vi "UDP_Stream(DMA).vi"() -> ()   [LabVIEW 2015]
uses:
  <vilib>/Platform/TimedLoop/XDataNode/timing_clust.ctl
  <vilib>/Platform/TimedLoop/XDataNode/nitl_modes.ctl
  <vilib>/Platform/TimedLoop/XDataNode/wakeup.ctl
  <vilib>/FPGAPlugInAG/cRIO-9063/niLvFpga_Open_cRIO-9063.vi
  <vilib>/rvi/interface/common/dynamic/niFpgaDynamicAddResources.vi
  <vilib>/Utility/error.llb/Error Cluster From Error Code.vi
  <vilib>/rvi/errors/niLvFpgaAdjustHostInterfaceError.vi
  <vilib>/Platform/TimedLoop/XDataNode/loadnilvce.vi
  <vilib>/rvi/interface/nirviOpenFPGA/nirviOpenFPGA.xnode
  FPGA Bitfiles/VCU-VEHICLEMODEL_FPGATarget_CANBasic(FPGA)_WVt1gIpoBPw.lvbitx
  Basic (FPGA) CAN Engine .vi
  <vilib>/rvi/interface/nirviReadWriteControl/nirviReadWriteControl.xnode
  <vilib>/Platform/TimedLoop/XDataNode/XDataNode.xnode
  <vilib>/Platform/TimedLoop/XDataNode/XDNodeRunTimeDep.lvlib
  NiFpgaLv.dll
  <vilib>/rvi/interface/Simulation/niFpgaSimulationCallBeginRW.vi
panel:
  out "Inbound Data String":string
  in  "Stop":bool
  out "CAN1 Data String":string
  out "CAN0 Data String":string
  out "CAN1-Time":u64
  out "CAN1-OldTime":u64
  out "CAN0-OldTime":u64
  out "CAN0-Time":u64
  in  "Start":bool
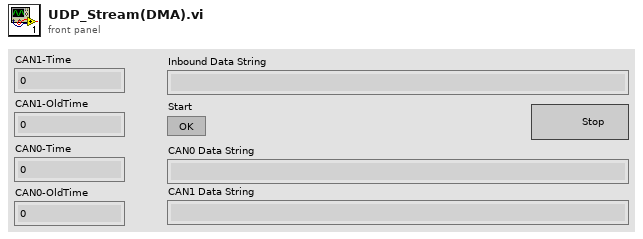
[diagram p1: front panel]
types:
  T1 = enum8{"Data Frame", "Remote Frame", "(reserved)", "(reserved) ", "(reserved)  ", "(reserved)   ", "Bus Error", "Transceiver Fault"}
  T2 = typedef "XDNodeRunTimeDep.lvlib/timing_clust.ctl" = cluster{"Expected End [f-1]":u64, "Actual End [f-1]":u64, "Finished Late? [f-1]":bool, "Expected End [i-1]":u64, "Actual End [i-1]":u64, "Finished Late? [i-1]":bool, "Expected Start [i]":u64, "Actual Start [i]":u64, "Expected Start [f]":u64, "Actual Start [f]":u64, "Source Name":string, "Structure Name":string, "Period":i64, "Deadline":i64, "Offset":i64, "Start":i64, "Priority":i32, "Timeout":i32, "Mode":T3, "Wakeup Reason":T4, "Error":errorcluster, "Source Type":string, "Secondary Source Type":string, "Global End Time":u64, "Global Start Time":u64, "Frame Duration":u64, "Iteration Duration":u64, "Assigned CPU":i32, "I/O Scan Engine Mode":u32}
  T3 = typedef "XDNodeRunTimeDep.lvlib/nitl_modes.ctl" = enum32{"No Change", "Process missed periods, maintain original phase", "Discard missed periods, maintain original phase", "Process missed periods, ignore original phase", "Discard missed periods, ignore original phase"}
  T4 = typedef "XDNodeRunTimeDep.lvlib/wakeup.ctl" = enum32{"Normal", "Aborted", "Asynchronous wakeup", "Timing source error", "Timed loop error", "Timeout"}
  T5 = cluster{u32, u32, u32, "type":enum8{"Data Frame", "Remote Frame", "(reserved)", "(reserved) ", "(reserved)  ", "(reserved)   ", "Bus Error", "Transceiver Fault"}, u8, u8, u8, u32[]}
  T6 = cluster{"timestamp high":u32, "timestamp low":u32, "identifier":u32, "type":enum8{"Data Frame", "Remote Frame", "(reserved)", "(reserved) ", "(reserved)  ", "(reserved)   ", "Bus Error", "Transceiver Fault"}, "info A":u8, "info B":u8, "data length":u8, "data":u8[]}
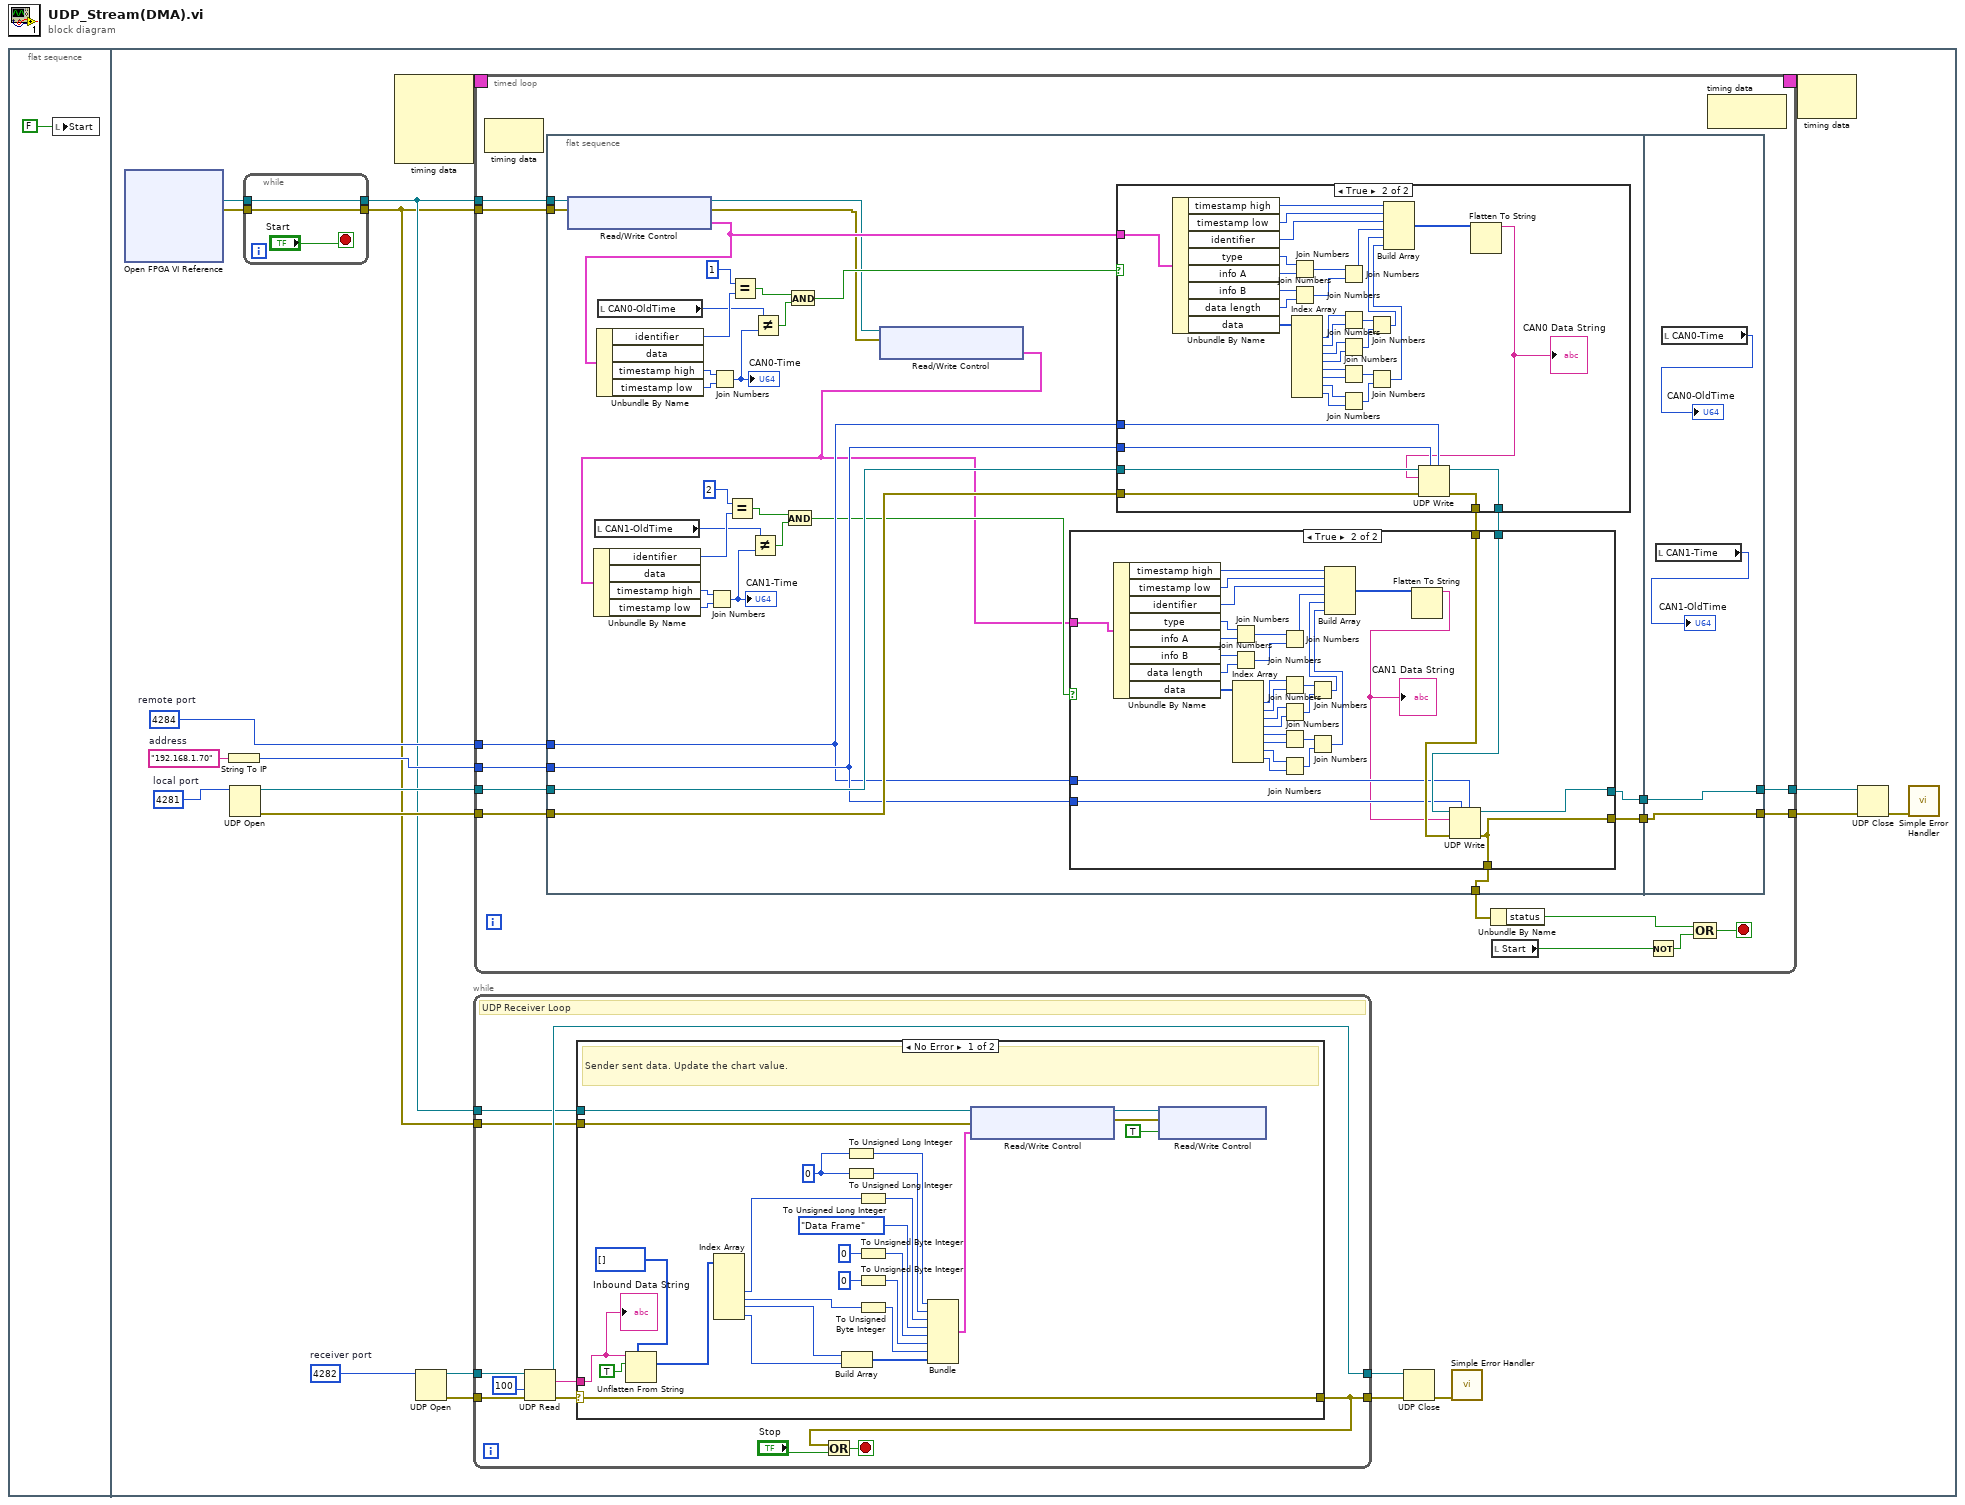
[diagram p0: block diagram]
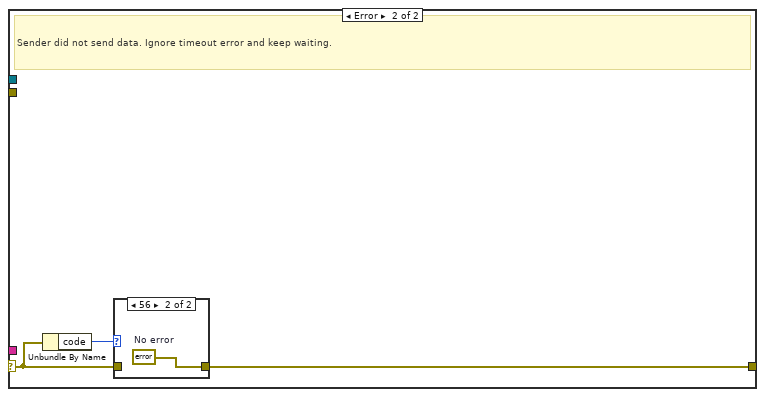
[diagram p2: hidden frame]
diagram:
  n1 = flat-sequence {
    frame #0 {
      n2 = local write "Start"(FALSE ("Stream")) -> ()
    }
    frame #1 {
      w4 = u16 4282  # receiver port
      w15 = u16 4284  # remote port
      w21 = u16 4281  # local port
      w22 = "192.168.1.70"  # address
      n3 = xnode "Open FPGA VI Reference"() -> ("FPGA VI Reference Out"=w19:refnum<k20>, "error out"=w18:errorcluster)  [unwired: 2 in]
      n4 = String To IP(1:w22) -> (0:w14:u32)
      n5 = UDP Open(11:w21) -> (port=w13:refnum<k16>, 0:w12:errorcluster)  [unwired: 4 in, 1 out]
      n6 = while {
        tunnel: [w194] -> w2
        tunnel: [w195] -> w3
        tunnel: w19 -> [w195]
        tunnel: w18 -> [w194]
        stop <- "Start" stop-if-true
      }
      n7 = node-c288() -> (w17:T2)  [unwired: 4 in]
      n8 = UDP Open(11:w4) -> (port=w5:refnum<k16>, 0:w6:errorcluster)  [unwired: 4 in, 1 out]
      n9 = while {
        tunnel: w5 -> [w33]
        tunnel: [w25] -> w9
        tunnel: w6 -> [w30]
        tunnel: [w26] -> w7
        tunnel: w3 -> [w24]
        tunnel: w2 -> [w23]
        stop <- w31 stop-if-true
        # "UDP Receiver Loop"
        n10 = UDP Read(connection ID=w33, timeout ms (25000)=100, 8:w30) -> (data out=w28:string, error out=w27:errorcluster, 3:w25:refnum<k16>)  [unwired: 3 out]
        n11 = case shown="No Error" w27 {
          selector: w27 -> [w59 w61]
          tunnel: w28 -> [w58 _]
          tunnel: [w59 w60] -> w26
          tunnel: w24 -> [w54 _]
          tunnel: w23 -> [w53 _]
          frame No Error {
            w42 = i16 0
            # "Sender sent data. Update the chart value."
            n12 = Unflatten From String(type=u32[] [], binary string=w58, data includes array or string size? (T)=TRUE) -> (value=w55:u32[])  [unwired: 2 in, 2 out]
            n13 = Index Array(array=w55) -> (element #3=w41:u32, element #4=w40:u32, element #5=w39:u32, element #6=w38:u32)  [unwired: 6 in, 2 out]
            n14 = Build Array(w39, w38) -> (w52:u32[])
            n15 = To Unsigned Long Integer(number=w42) -> (unsigned 32bit integer=w45:u32)
            n16 = To Unsigned Long Integer(number=w42) -> (unsigned 32bit integer=w46:u32)
            n17 = To Unsigned Long Integer(number=w41) -> (unsigned 32bit integer=w47:u32)
            n18 = To Unsigned Byte Integer(number=u8 0 ("info A")) -> (unsigned 8bit integer=w48:u8)
            n19 = To Unsigned Byte Integer(number=u8 0 ("info B")) -> (unsigned 8bit integer=w49:u8)
            n20 = To Unsigned Byte Integer(number=w40) -> (unsigned 8bit integer=w50:u8)
            n21 = Bundle(w45, w46, w47, "type"=T1."Data Frame", w48, w49, w50, w52) -> (w37:T5)  [unwired: 1 in]
            n22 = xnode "Read/Write Control"("FPGA VI Reference In"=w54, "error in"=w53, "CAN0 - Transmit Frame"=w37) -> ("FPGA VI Reference Out"=w35:refnum<k20>, "error out"=w34:errorcluster)
            n23 = xnode "Read/Write Control"("FPGA VI Reference In"=w35, "error in"=w34, "CAN0 - Transmit"=TRUE) -> ()  [unwired: 2 out]
            "Inbound Data String" <- w58
          }
          frame Error {
            # "Sender did not send data. Ignore timeout error and keep waiting."
            n24 = Unbundle By Name(w61) -> ("code"=w62:i32)
            n25 = case shown="56" w62 {
              tunnel: w61 -> [w63 _]
              tunnel: [w63 w64] -> w60
              frame Default {
              }
              frame 56 {
                w64 = errorcluster {"status"=FALSE, "code"=0, "source"=""}  # No error
              }
            }
          }
        }
        n26 = Or(x=w26, y="Stop") -> (x .or. y?=w31:bool)
      }
      n27 = timed-loop {
        timing: w17 -> [_]
        timing-out: [_] -> w16
        tunnel: w3 -> [w79]
        tunnel: w2 -> [w78]
        tunnel: w15 -> [w72]
        tunnel: w14 -> [w73]
        tunnel: w13 -> [w71]
        tunnel: w12 -> [w70]
        tunnel: [w68] -> w11
        tunnel: [w69] -> w10
        stop <- w74 stop-if-true
        n28 = node-c288() -> ()  [unwired: 1 in, 1 out]
        n29 = flat-sequence {
          tunnel: w79 -> [w104]
          tunnel: w78 -> [w103]
          tunnel: w73 -> [w87]
          tunnel: w72 -> [w86]
          tunnel: w71 -> [w102]
          tunnel: w70 -> [w100]
          tunnel: [w89] -> w67
          tunnel: [w83] -> w66
          tunnel: [w82] -> w65
          tunnel: [w186] -> w68
          tunnel: [w187] -> w69
          tunnel: w66 -> [w187]
          tunnel: w65 -> [w186]
          frame #0 {
            n30 = xnode "Read/Write Control"("FPGA VI Reference In"=w104, "error in"=w103) -> ("FPGA VI Reference Out"=w81:refnum<k20>, "error out"=w80:errorcluster, "CAN0 - Received Frame"=w101:T6)
            n31 = local read "CAN1-OldTime"() -> (w95:u64)
            n32 = Unbundle By Name(w101) -> ("identifier"=w111:u32, "timestamp high"=w110:u32, "timestamp low"=w109:u32)  [unwired: 1 out]
            n33 = local read "CAN0-OldTime"() -> (w108:u64)
            n34 = Join Numbers(hi=w110, lo=w109) -> ((hi.lo)=w107:u64)
            "CAN0-Time" <- w107
            n35 = Equal?(x=u32 1, y=w111) -> (x = y?=w106:bool)
            n36 = Not Equal?(x=w108, y=w107) -> (x != y?=w105:bool)
            n37 = And(x=w106, y=w105) -> (x .and. y?=w91:bool)
            n38 = xnode "Read/Write Control"("FPGA VI Reference In"=w81, "error in"=w80) -> ("CAN1 - Received Frame"=w84:T6)  [unwired: 2 out]
            n39 = Unbundle By Name(w84) -> ("identifier"=w98:u32, "timestamp high"=w97:u32, "timestamp low"=w96:u32)  [unwired: 1 out]
            n40 = Join Numbers(hi=w97, lo=w96) -> ((hi.lo)=w94:u64)
            "CAN1-Time" <- w94
            n41 = Equal?(x=u32 2, y=w98) -> (x = y?=w93:bool)
            n42 = Not Equal?(x=w95, y=w94) -> (x != y?=w92:bool)
            n43 = And(x=w93, y=w92) -> (x .and. y?=w85:bool)
            n44 = case shown="True" w91 {
              tunnel: w87 -> [_ w184]
              tunnel: w86 -> [_ w183]
              tunnel: w102 -> [w150 w182]
              tunnel: [w149 w152] -> w90
              tunnel: w101 -> [_ w155]
              tunnel: w100 -> [w149 w153]
              tunnel: [w150 w151] -> w88
              frame False {
              }
              frame True {
                n45 = Unbundle By Name(w155) -> ("timestamp high"=w175:u32, "timestamp low"=w176:u32, "identifier"=w177:u32, "type"=w158:T1, "info A"=w157:u8, "info B"=w159:u8, "data length"=w160:u8, "data"=w162:u8[])
                n46 = Join Numbers(hi=w158, lo=w157) -> ((hi.lo)=w161:u16)
                n47 = Join Numbers(hi=w159, lo=w160) -> ((hi.lo)=w156:u16)
                n48 = Index Array(array=w162) -> (element #1=w163:u8, element #2=w164:u8, element #3=w165:u8, element #4=w166:u8, element #5=w167:u8, element #6=w168:u8, element #7=w169:u8, element #8=w170:u8)  [unwired: 8 in]
                n49 = Join Numbers(hi=w161, lo=w156) -> ((hi.lo)=w178:u32)
                n50 = Join Numbers(hi=w163, lo=w164) -> ((hi.lo)=w171:u16)
                n51 = Join Numbers(hi=w165, lo=w166) -> ((hi.lo)=w172:u16)
                n52 = Join Numbers(hi=w167, lo=w168) -> ((hi.lo)=w173:u16)
                n53 = Join Numbers(hi=w169, lo=w170) -> ((hi.lo)=w174:u16)
                n54 = Join Numbers(hi=w171, lo=w172) -> ((hi.lo)=w179:u32)
                n55 = Join Numbers(hi=w173, lo=w174) -> ((hi.lo)=w180:u32)
                n56 = Build Array(w175, w176, w177, w178, w179, w180) -> (w154:u32[])
                n57 = Flatten To String(anything=w154) -> (data string=w181:string)  [unwired: 3 in, 2 out]
                "CAN0 Data String" <- w181
                n58 = UDP Write(address=w184, port or service name=w183, connection ID=w182, data in=w181, 8:w153) -> (error out=w152:errorcluster, 3:w151:refnum<k16>)  [unwired: 1 in]
              }
            }
            n59 = case shown="True" w85 {
              tunnel: w90 -> [w114 w148]
              tunnel: [w114 w116] -> w89
              tunnel: w88 -> [w113 w147]
              tunnel: w87 -> [_ w146]
              tunnel: w86 -> [_ w145]
              tunnel: w84 -> [_ w118]
              tunnel: [w113 w117] -> w83
              tunnel: [w114 w116] -> w82
              frame False {
              }
              frame True {
                n60 = Unbundle By Name(w118) -> ("timestamp high"=w124:u32, "timestamp low"=w123:u32, "identifier"=w122:u32, "type"=w141:T1, "info A"=w142:u8, "info B"=w140:u8, "data length"=w139:u8, "data"=w137:u8[])
                n61 = Join Numbers(hi=w141, lo=w142) -> ((hi.lo)=w138:u16)
                n62 = Join Numbers(hi=w140, lo=w139) -> ((hi.lo)=w143:u16)
                n63 = Index Array(array=w137) -> (element #1=w136:u8, element #2=w135:u8, element #3=w134:u8, element #4=w133:u8, element #5=w132:u8, element #6=w131:u8, element #7=w130:u8, element #8=w129:u8)  [unwired: 8 in]
                n64 = Join Numbers(hi=w138, lo=w143) -> ((hi.lo)=w121:u32)
                n65 = Join Numbers(hi=w136, lo=w135) -> ((hi.lo)=w128:u16)
                n66 = Join Numbers(hi=w134, lo=w133) -> ((hi.lo)=w127:u16)
                n67 = Join Numbers(hi=w132, lo=w131) -> ((hi.lo)=w126:u16)
                n68 = Join Numbers(hi=w130, lo=w129) -> ((hi.lo)=w125:u16)
                n69 = Join Numbers(hi=w128, lo=w127) -> ((hi.lo)=w120:u32)
                n70 = Join Numbers(hi=w126, lo=w125) -> ((hi.lo)=w119:u32)
                n71 = Build Array(w124, w123, w122, w121, w120, w119) -> (w144:u32[])
                n72 = Flatten To String(anything=w144) -> (data string=w115:string)  [unwired: 3 in, 2 out]
                "CAN1 Data String" <- w115
                n73 = UDP Write(address=w146, port or service name=w145, connection ID=w147, data in=w115, 8:w148) -> (error out=w116:errorcluster, 3:w117:refnum<k16>)  [unwired: 1 in]
              }
            }
          }
          frame #1 {
            n74 = local read "CAN1-Time"() -> (→"CAN1-OldTime":u64)
            n75 = local read "CAN0-Time"() -> (→"CAN0-OldTime":u64)
          }
        }
        n76 = Unbundle By Name(w67) -> ("status"=w75:bool)
        n77 = local read "Start"() -> (w76:bool)
        n78 = Not(x=w76) -> (.not. x?=w77:bool)
        n79 = Compound Arithmetic op=OR(w75, w77) -> (w74:bool)
        n80 = node-c288() -> ()  [unwired: 1 in, 1 out]
      }
      n81 = UDP Close(connection ID=w9, 8:w7) -> (error out=w8:errorcluster)  [unwired: 1 out]
      n82 = call <vilib>:"Simple Error Handler.vi"("error in (no error)"=w8) -> ()  [unwired: 1 in, 8 out]
      n83 = node-c288(w16) -> ()  [unwired: 1 out]
      n84 = UDP Close(connection ID=w10, 8:w11) -> (error out=w20:errorcluster)  [unwired: 1 out]
      n85 = call <vilib>:"Simple Error Handler.vi"("error in (no error)"=w20) -> ()  [unwired: 4 in, 5 out]
    }
  }
